vi "Synergy VI.vi"(0 "Wrist X to graph":dbl[](array[numeric]), 5 "Wrist X Tags":i32[](array[numeric]), 7 "Wrist X to derivate":dbl[](array[numeric]), 9 "Shoulder X to derivate":dbl[](array[numeric]), 11 "Shoulder X":dbl[](array[numeric])) -> (4 "same direction %":i32, 6 "opposite direction %":i32, 8 "WristX-ShouldeX graph":i32[](array[numeric]))   [LabVIEW 2020]
uses:
  <vilib>/Analysis/NI_AALPro.lvlib
panel:
  out "opposite direction":i32
  out "same direction":i32
  # "Outputs"
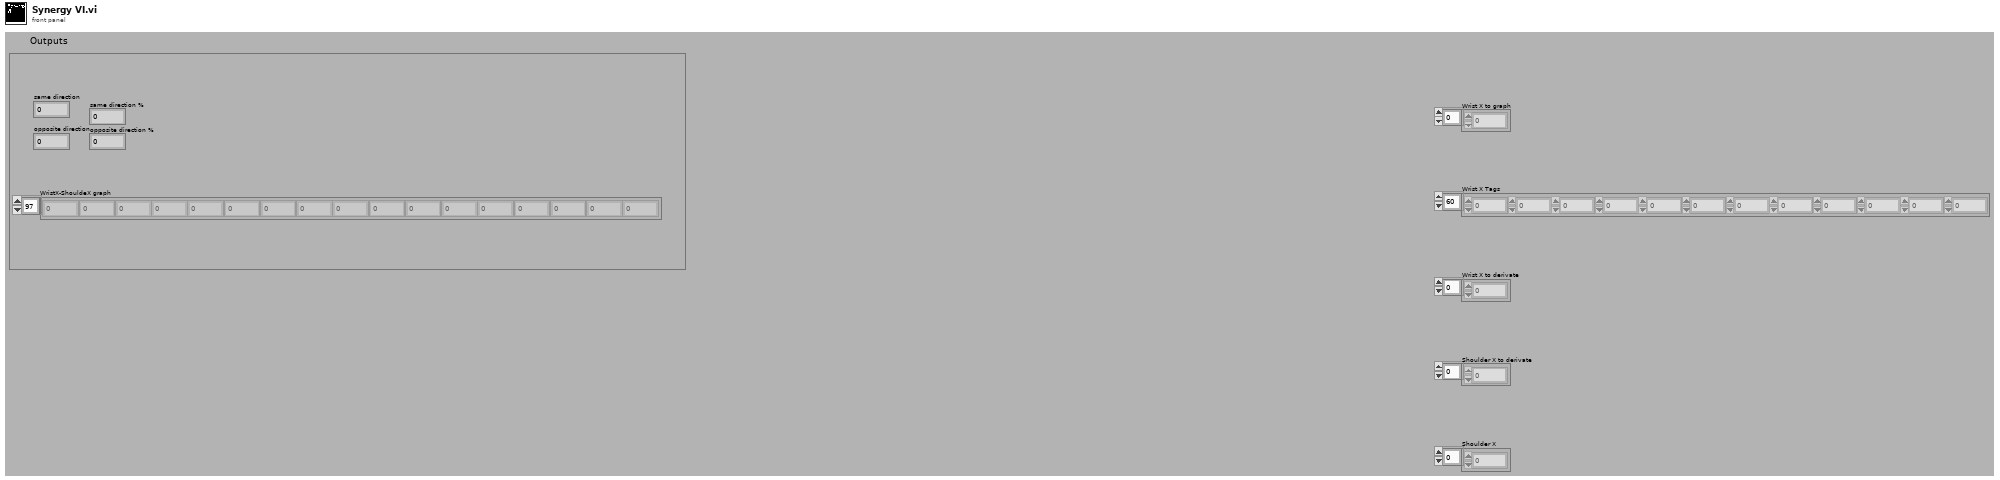
[diagram p1: front panel]
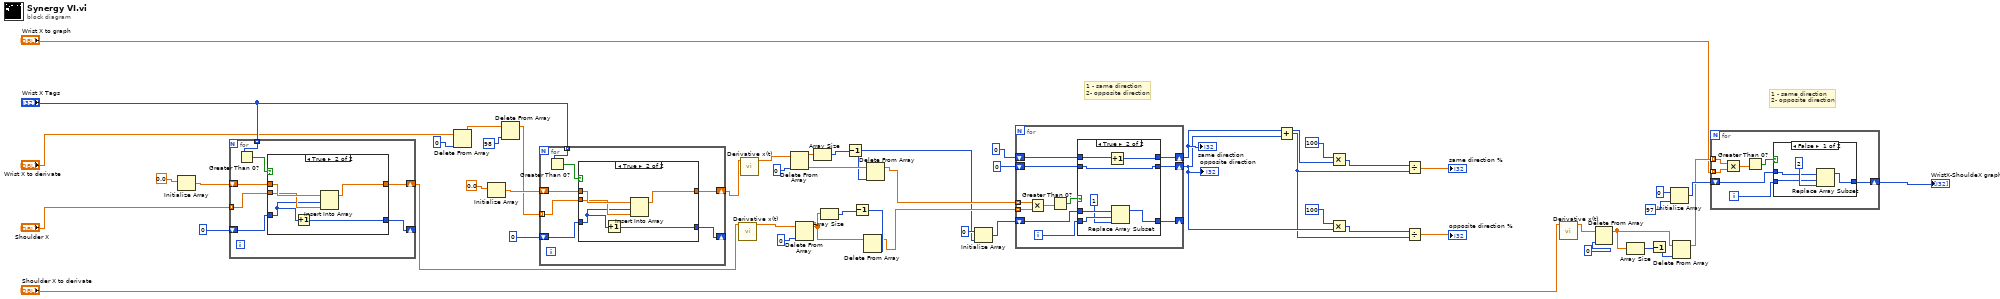
[diagram p0: block diagram]
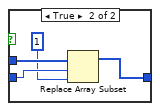
[diagram p2: hidden frame]
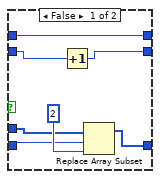
[diagram p3: hidden frame]
diagram:
  # "1 - same direction\n2- opposite direction"
  # "1 - same direction\n2- opposite direction"
  n1 = Initialize Array(0.0) -> (w52:dbl[])  [unwired: 1 in]
  n2 = for {
    tunnel: "Wrist X Tags" -> [w57] mode=indexing
    shift-right: [w55] -> w36
    shift-left: w52 -> [w56]
    tunnel: "Shoulder X" -> [w58] mode=indexing
    shift-right: [w53] -> _
    shift-left: 0 -> [w54]
    n3 = Greater Than 0?(x=w57) -> (x > 0?=w59:bool)
    n4 = case shown="True" w59 {
      tunnel: w58 -> [_ w65]
      tunnel: w56 -> [w61 w66]
      tunnel: [w61 w64] -> w55
      tunnel: w54 -> [w60 w63]
      tunnel: [w60 w62] -> w53
      frame False {
      }
      frame True {
        n5 = Increment(x=w63) -> (x+1=w62:i32)
        n6 = Insert Into Array(array=w66, index=w63, new element=w65) -> (w64:dbl[])
      }
    }
  }
  n7 = Delete From Array(array="Wrist X to derivate", index=0) -> (array with subset deleted=w45:dbl[])  [unwired: 1 in, 1 out]
  n8 = Initialize Array(0.0) -> (w49:dbl[])  [unwired: 1 in]
  n9 = Delete From Array(array=w45, index=98) -> (array with subset deleted=w43:dbl[])  [unwired: 1 in, 1 out]
  n10 = for {
    tunnel: "Wrist X Tags" -> [w71] mode=indexing
    shift-right: [w69] -> w38
    shift-left: w49 -> [w70]
    tunnel: w43 -> [w72] mode=indexing
    shift-right: [w67] -> _
    shift-left: 0 -> [w68]
    n11 = Greater Than 0?(x=w71) -> (x > 0?=w73:bool)
    n12 = case shown="True" w73 {
      tunnel: w72 -> [_ w79]
      tunnel: w70 -> [w75 w80]
      tunnel: [w75 w78] -> w69
      tunnel: w68 -> [w74 w77]
      tunnel: [w74 w76] -> w67
      frame False {
      }
      frame True {
        n13 = Increment(x=w77) -> (x+1=w76:i32)
        n14 = Insert Into Array(array=w80, index=w77, new element=w79) -> (w78:dbl[])
      }
    }
  }
  n15 = call <vilib>:"Derivative x(t).vi"("X"=w36) -> ("dX/dt"=w39:dbl[])  [unwired: 9 in, 1 out]
  n16 = call <vilib>:"Derivative x(t).vi"("X"=w38) -> ("dX/dt"=w41:dbl[])  [unwired: 9 in, 1 out]
  n17 = Delete From Array(array=w41, index=0) -> (array with subset deleted=w37:dbl[])  [unwired: 1 in, 1 out]
  n18 = Delete From Array(array=w39, index=0) -> (array with subset deleted=w34:dbl[])  [unwired: 1 in, 1 out]
  n19 = Array Size(array=w37) -> (size(s)=w28:i32)
  n20 = Array Size(array=w34) -> (size(s)=w35:i32)
  n21 = Decrement(x=w28) -> (x-1=w27:i32)
  n22 = Decrement(x=w35) -> (x-1=w33:i32)
  n23 = Delete From Array(array=w34, index=w33) -> (array with subset deleted=w29:dbl[])  [unwired: 1 in, 1 out]
  n24 = Delete From Array(array=w37, index=w27) -> (array with subset deleted=w30:dbl[])  [unwired: 1 in, 1 out]
  n25 = Initialize Array(0, w27) -> (w31:i32[])
  n26 = for {
    tunnel: w30 -> [w91] mode=indexing
    tunnel: w29 -> [w90] mode=indexing
    shift-right: [w87] -> _
    shift-left: w31 -> [w86]
    shift-right: [w83] -> w19
    shift-left: 0 -> [w84]
    shift-right: [w81] -> w23
    shift-left: 0 -> [w82]
    i -> [w88]
    n27 = Multiply(x=w91, y=w90) -> (x*y=w89:dbl)
    n28 = Greater Than 0?(x=w89) -> (x > 0?=w85:bool)
    n29 = case shown="True" w85 {
      tunnel: w88 -> [w96 w103]
      tunnel: [w95 w105] -> w87
      tunnel: w86 -> [w97 w104]
      tunnel: w84 -> [w94 w99]
      tunnel: [w93 w99] -> w83
      tunnel: w82 -> [w92 w101]
      tunnel: [w92 w100] -> w81
      frame False {
        n30 = Increment(x=w94) -> (x+1=w93:i32)
        n31 = Replace Array Subset(array=w97, new element=2, index=w96) -> (w95:i32[])
      }
      frame True {
        n32 = Increment(x=w101) -> (x+1=w100:i32)
        n33 = Replace Array Subset(array=w104, new element=1, index=w103) -> (w105:i32[])
      }
    }
  }
  "same direction" <- w23
  "opposite direction" <- w19
  n34 = Add(x=w23, y=w19) -> (x+y=w18:i32)
  n35 = Multiply(x=100, y=w23) -> (x*y=w22:i32)
  n36 = Multiply(x=100, y=w19) -> (x*y=w20:i32)
  n37 = Divide(x=w22, y=w18) -> (x/y=→"same direction %":dbl)
  n38 = Divide(x=w20, y=w18) -> (x/y=→"opposite direction %":dbl)
  n39 = call <vilib>:"Derivative x(t).vi"("X"="Shoulder X to derivate") -> ("dX/dt"=w14:dbl[])  [unwired: 9 in, 1 out]
  n40 = Delete From Array(array=w14, index=0) -> (array with subset deleted=w12:dbl[])  [unwired: 1 in, 1 out]
  n41 = Array Size(array=w12) -> (size(s)=w13:i32)
  n42 = Decrement(x=w13) -> (x-1=w11:i32)
  n43 = Initialize Array(0, 97) -> (w16:i32[])
  n44 = Delete From Array(array=w12, index=w11) -> (array with subset deleted=w10:dbl[])  [unwired: 1 in, 1 out]
  n45 = for {
    shift-right: [w110] -> w6
    shift-left: w16 -> [w109]
    tunnel: w10 -> [w107] mode=indexing
    tunnel: "Wrist X to graph" -> [w106] mode=indexing
    i -> [w111]
    n46 = Multiply(x=w107, y=w106) -> (x*y=w112:dbl)
    n47 = Greater Than 0?(x=w112) -> (x > 0?=w108:bool)
    n48 = case shown="False" w108 {
      tunnel: w111 -> [w114 w118]
      tunnel: [w113 w120] -> w110
      tunnel: w109 -> [w115 w119]
      frame False {
        n49 = Replace Array Subset(array=w115, new element=2, index=w114) -> (w113:i32[])
      }
      frame True {
        n50 = Replace Array Subset(array=w119, new element=1, index=w118) -> (w120:i32[])
      }
    }
  }
  "WristX-ShouldeX graph" <- w6
